vi "Choosed_Options_to_Array.vi"(8 "error in (no error)":errorcluster, 11 "UI_Cluster_In":T1) -> (0 "error out":errorcluster, 3 "UI_Cluster_Out":T1)   [LabVIEW 2020]
uses:
  controls/UI_Ref_Cluster.ctl
  07e20563-7f03-42b7-a7af-6da6fdcb7415.vi
  <vilib>/Comparison/Less/Less Functor/Less Functor.lvclass
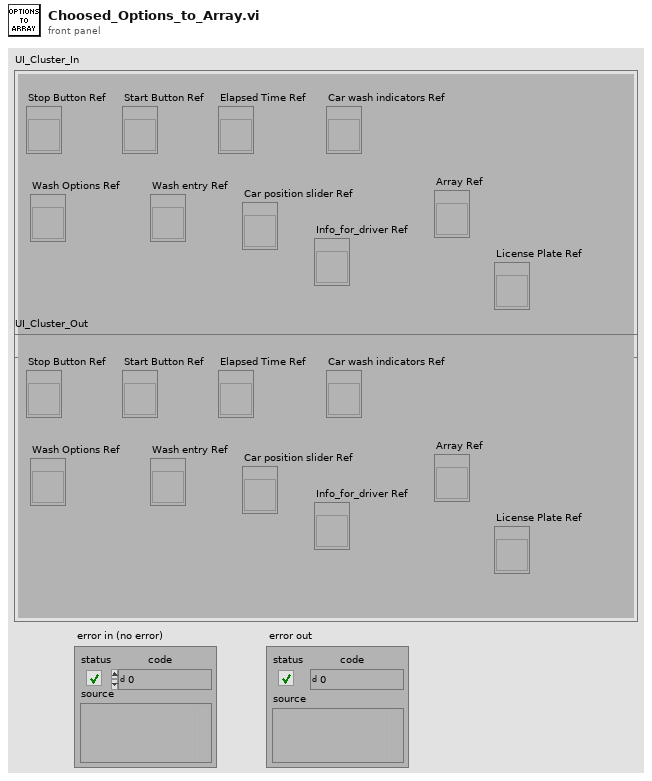
[diagram p1: front panel]
types:
  T1 = typedef "UI_Ref_Cluster.ctl" = cluster{"Stop Button Ref":refnum<vi>, "Start Button Ref":refnum<vi>, "Elapsed Time Ref":refnum<vi>, "Car wash indicators Ref":refnum<vi>, "Wash Options Ref":refnum<vi>, "Wash entry Ref":refnum<vi>, "Car position slider Ref":refnum<vi>, "Info_for_driver Ref":refnum<vi>, "Array Ref":refnum<vi>, "License Plate Ref":refnum<vi>}
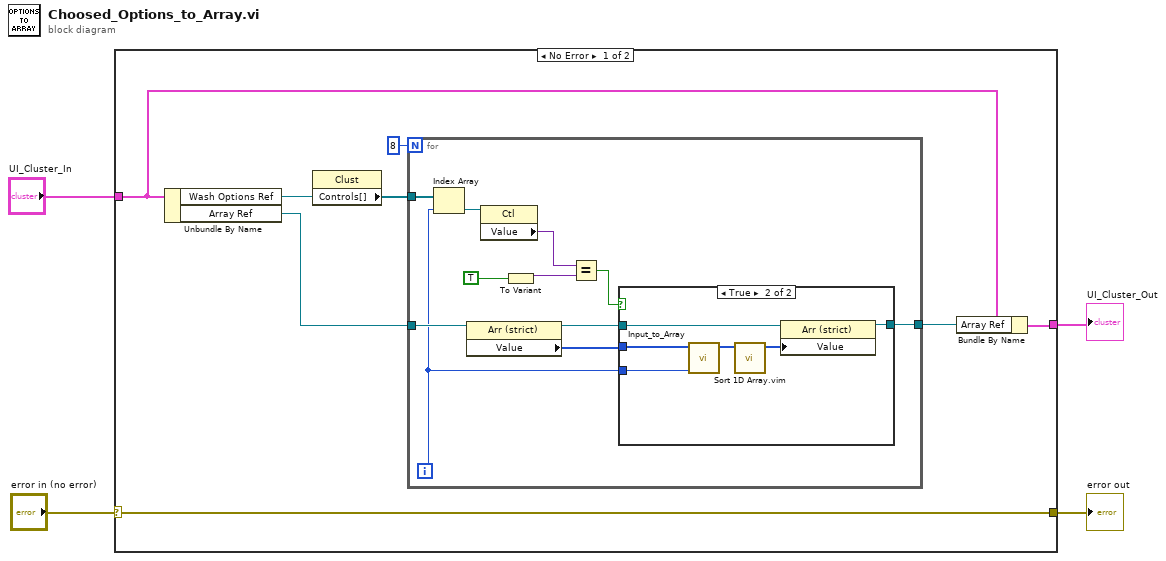
[diagram p0: block diagram]
diagram:
  n1 = case shown="No Error" "error in (no error)" {
    selector: "error in (no error)" -> [w7 w32]
    tunnel: [w7 w32] -> w3
    tunnel: "UI_Cluster_In" -> [w8 w31]
    tunnel: [w6 w31] -> w1
    frame No Error {
      n2 = Unbundle By Name(w8) -> ("Wash Options Ref"=w12:refnum<vi>, "Array Ref"=w9:refnum<vi>)
      n3 = property class="Clust"(reference=w12) -> ("Controls[]"=w10:refnum<vi>[])  [unwired: 1 in, 2 out]
      n4 = for {
        N: 8 -> [_]
        tunnel: w10 -> [w23]
        tunnel: w9 -> [w18]
        tunnel: [w14] -> w5
        i -> [w16]
        n5 = Index Array(array=w23, index=w16) -> (element=w22:refnum<vi>)
        n6 = property class="Arr (strict)"(reference=w18) -> (reference out=w15:refnum<vi>, "Value"=w17:i8[])  [unwired: 1 in, 1 out]
        n7 = property class="Ctl"(reference=w22) -> ("Value"=w21:variant)  [unwired: 1 in, 2 out]
        n8 = To Variant(anything=TRUE) -> (Variant=w13:variant)
        n9 = Equal?(x=w21, y=w13) -> (x = y?=w19:bool)
        n10 = case shown="True" w19 {
          tunnel: w17 -> [_ w29]
          tunnel: w16 -> [_ w28]
          tunnel: w15 -> [w24 w27]
          tunnel: [w24 w26] -> w14
          frame False {
          }
          frame True {
            n11 = call "Input_to_Array.vi"("Numeric"=w28, "Array_In"=w29) -> ("Array_Out"=w30:i8[])  [unwired: 9 in]
            n12 = call "Sort 1D Array.vim"("unsorted array"=w30) -> ("sorted array"=w25:i8[])  [unwired: 10 in]
            n13 = property class="Arr (strict)"(reference=w27, "Value"=w25) -> (reference out=w26:refnum<vi>)  [unwired: 1 in, 1 out]
          }
        }
      }
      n14 = Bundle By Name(cluster=w8, "Array Ref"=w5) -> (w6:T1)
    }
    frame Error {
    }
  }
  "UI_Cluster_Out" <- w1
  "error out" <- w3
